vi "HDF5_append-dataset-Test6vi.vi"() -> ()   [LabVIEW 2018]
uses:
  <vilib>/addons/h5labview2/file/H5F.lvlib
  <vilib>/addons/h5labview2/file/H5Fmode.ctl
  <vilib>/addons/h5labview2/dataset/H5D.lvlib
  HDF5/HDF5_ToneInfoClust.ctl
  <vilib>/addons/h5labview2/dataset/H5Dwrite.llb/H5Dwrite.xnode
  <vilib>/addons/h5labview2/space/H5S.lvlib
  <vilib>/addons/h5labview2/base/H5Equery.vi
  HDF5/lib_path_mod_20200519.vi
  <vilib>/addons/h5labview2/dataset/H5Dread.llb/H5Dread.xnode
  HDF5/HDF5_ToneInfoZoomAryClust.ctl
  <vilib>/addons/h5labview2/base/hid_t_renamed.ctl
panel:
  out "Tone2":T1[](array[typedef])
  out "Tone1":T1[](array[typedef])
  in  "data":i32[][](array[numeric])=[[0, 1, 2, 3, 4], [5, 6, 7, 8, 9]]
  out "ms/append":dbl
  out "timer (ms)":u32
  out "progress":i32(slide)=9999 scale=0.0..10000.0
  in  "repetitions":i32=10
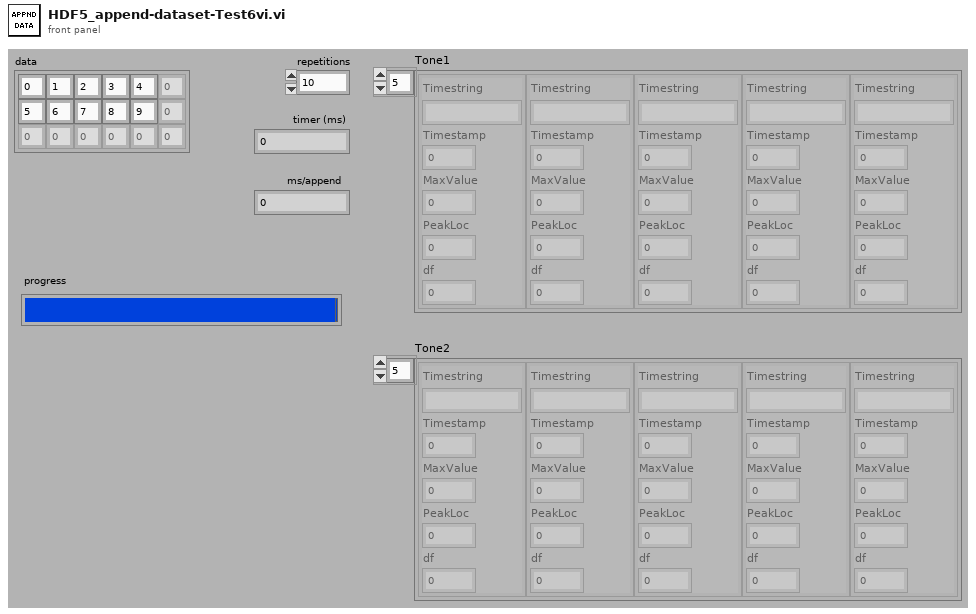
[diagram p1: front panel]
types:
  T1 = typedef "HDF5_ToneInfoClust.ctl" = cluster{"Timestring":string, "Timestamp":dbl, "MaxValue":dbl, "PeakLoc":dbl, "df":dbl}
  T2 = typedef "H5F.lvlib/H5Fmode.ctl" = enum16{"read-only", "read-write", "overwrite", "create new", "open or create"}
  T3 = typedef "HDF5_ToneInfoZoomAryClust.ctl" = cluster{"Timestring":string, "Timestamp":timestamp, "MaxValue":dbl, "PeakLoc":dbl, "df":dbl, "Zoom":dbl[]}
  T4 = typedef "HDF5_ToneInfoClust.ctl" = cluster{"Timestring":string, "Timestamp":timestamp, "MaxValue":dbl, "PeakLoc":dbl, "df":dbl}
  T5 = typedef "hid_t.ctl" = i32
  T6 = typedef "hid_t_renamed.ctl" = i32
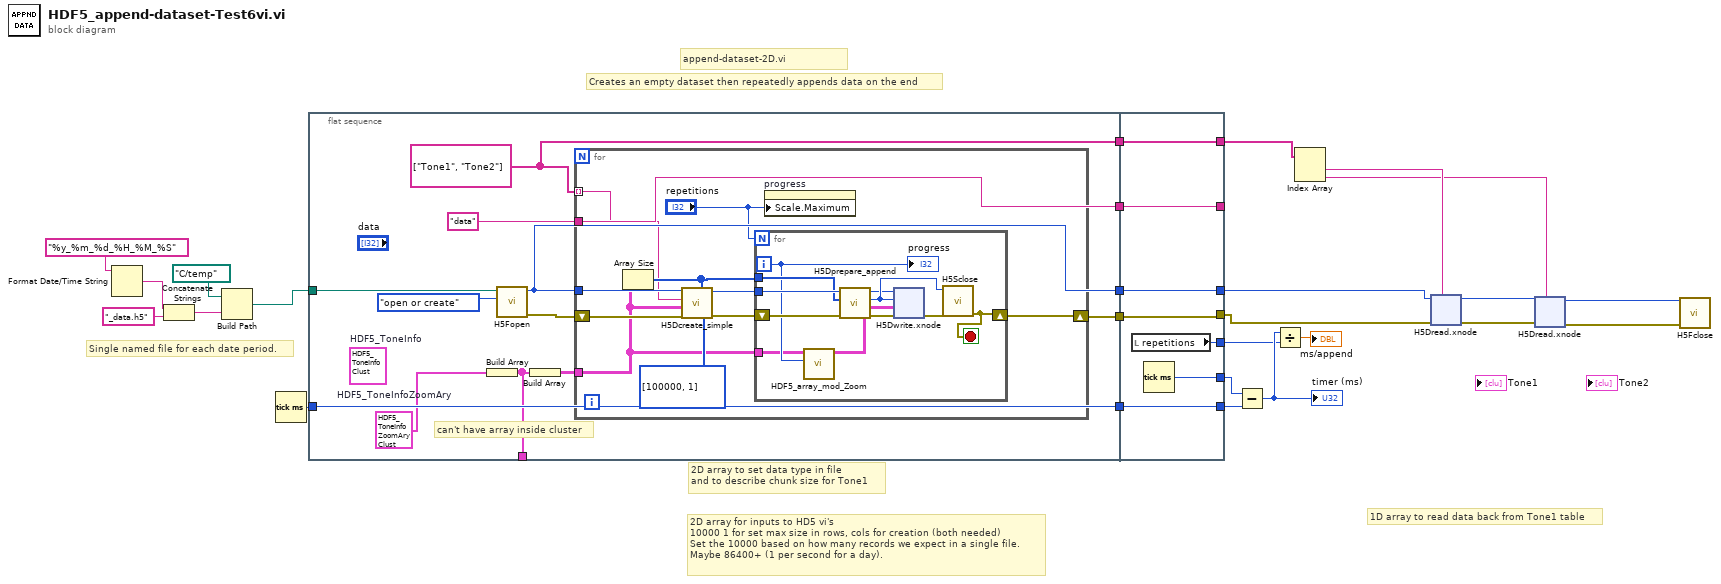
[diagram p0: block diagram]
diagram:
  # "2D array to set data type in file\nand to describe chunk size for Tone1"
  # "1D array to read data back from Tone1 table"
  # "2D array for inputs to HD5 vi's\n10000 1 for set max size in rows, cols for creation (both needed) \nSet the 10000 based on how many records we expect in a single file.\nMaybe 86400+ (1 per second for a day)."
  # "Single named file for each date period."
  # "Creates an empty dataset then repeatedly appends data on the end"
  # "append-dataset-2D.vi"
  n1 = Format Date/Time String(time format string (%c)="%y_%m_%d_%H_%M_%S") -> (date/time string=w17:string)  [unwired: 2 in]
  n2 = Concatenate Strings(w17, "_data.h5" ("string")) -> (w19:string)
  n3 = Build Path(base path=path "C:/temp", name or relative path=w19) -> (appended path=w15:path)
  n4 = Tick Count (ms)() -> (millisecond timer value=w27:u32)
  n5 = flat-sequence {
    tunnel: w27 -> [w36]
    tunnel: [w36] -> w26
    tunnel: w15 -> [w35]
    tunnel: [w33] -> w13
    tunnel: [w32] -> w12
    tunnel: [w31] -> w1
    tunnel: [w30] -> w11
    tunnel: [w29] -> w9
    tunnel: w26 -> [w84]
    tunnel: [w85] -> w25
    tunnel: [w84] -> w24
    tunnel: [w83] -> w22
    tunnel: [w82] -> w14
    tunnel: w13 -> [w82]
    tunnel: [w81] -> _
    tunnel: w12 -> [w81]
    tunnel: [w80] -> w10
    tunnel: w11 -> [w80]
    tunnel: w9 -> [w79]
    tunnel: [w79] -> w7
    frame #0 {
      w28 = T3 {"Timestring"="Timestamp string goes here", "Timestamp"=timestamp(0 s since 1904-01-01), "MaxValue"=0.0, "PeakLoc"=0.0, "df"=0.0, "Zoom"=[0.0, 0.0, 0.0, 0.0, 0.0, 0.0, 0.0, 0.0, 0.0, 0.0, 0.0, 0.0, 0.0, 0.0, 0.0, 0.0, 0.0, 0.0, 0.0, 0.0, 0.0, 0.0, 0.0, 0.0, 0.0, 0.0, 0.0, 0.0, 0.0, 0.0, 0.0, 0.0, 0.0, 0.0, 0.0, 0.0, 0.0, 0.0, 0.0, 0.0, 0.0, 0.0, 0.0, 0.0, 0.0, 0.0, 0.0, 0.0, 0.0, 0.0, 0.0, 0.0, 0.0, 0.0, 0.0, 0.0, 0.0, 0.0, 0.0, 0.0, 0.0, 0.0, 0.0, 0.0, 0.0, 0.0, 0.0, 0.0, 0.0, 0.0, 0.0, 0.0, 0.0, 0.0, 0.0, 0.0, 0.0, 0.0, 0.0, 0.0, 0.0, 0.0, 0.0, 0.0, 0.0, 0.0, 0.0, 0.0, 0.0, 0.0, 0.0, 0.0, 0.0, 0.0, 0.0, 0.0, 0.0, 0.0, 0.0, 0.0, 0.0, 0.0, 0.0, 0.0, 0.0, 0.0, 0.0, 0.0, 0.0, 0.0, 0.0, 0.0, 0.0, 0.0, 0.0, 0.0, 0.0, 0.0, 0.0, 0.0, 0.0, 0.0, 0.0, 0.0, 0.0, 0.0, 0.0, 0.0, 0.0, 0.0, 0.0, 0.0, 0.0, 0.0, 0.0, 0.0, 0.0, 0.0, 0.0, 0.0, 0.0, 0.0, 0.0, 0.0, 0.0, 0.0, 0.0, 0.0, 0.0, 0.0, 0.0, 0.0, 0.0, 0.0, 0.0, 0.0, 0.0, 0.0, 0.0, 0.0, 0.0, 0.0, 0.0, 0.0, 0.0, 0.0, 0.0, 0.0, 0.0, 0.0, 0.0, 0.0, 0.0, 0.0, 0.0, 0.0, 0.0, 0.0, 0.0, 0.0, 0.0, 0.0, 0.0, 0.0, 0.0, 0.0, 0.0, 0.0, 0.0, 0.0, 0.0, 0.0, 0.0, 0.0, 0.0, 0.0, 0.0, 0.0, 0.0, 0.0, 0.0, 0.0, 0.0, 0.0, 0.0, 0.0, 0.0, 0.0, 0.0, 0.0, 0.0, 0.0, 0.0, 0.0, 0.0, 0.0, 0.0, 0.0, 0.0, 0.0, 0.0, 0.0, 0.0, 0.0, 0.0, 0.0, 0.0, 0.0, 0.0, 0.0, 0.0, 0.0, 0.0, 0.0, 0.0, 0.0, 0.0, 0.0, 0.0, 0.0, 0.0, 0.0, 0.0, 0.0, 0.0, 0.0, 0.0, 0.0, 0.0, 0.0, 0.0, 0.0, 0.0, 0.0, 0.0, 0.0, 0.0, 0.0, 0.0, 0.0, 0.0, 0.0, 0.0, 0.0, 0.0, 0.0, 0.0, 0.0, 0.0, 0.0, 0.0, 0.0, 0.0, 0.0, 0.0, 0.0, 0.0, 0.0, 0.0, 0.0, 0.0, 0.0, 0.0, 0.0, 0.0, 0.0, 0.0, 0.0, 0.0, 0.0, 0.0, 0.0, 0.0, 0.0, 0.0, 0.0, 0.0, 0.0, 0.0, 0.0, 0.0, 0.0, 0.0, 0.0, 0.0, 0.0, 0.0, 0.0, 0.0, 0.0, 0.0, 0.0, 0.0, 0.0, 0.0, 0.0, 0.0, 0.0, 0.0, 0.0, 0.0, 0.0, 0.0, 0.0, 0.0, 0.0, 0.0, 0.0, 0.0, 0.0, 0.0, 0.0, 0.0, 0.0, 0.0, 0.0, 0.0, 0.0, 0.0, 0.0, 0.0, 0.0, 0.0, 0.0, 0.0, 0.0, 0.0, 0.0, 0.0, 0.0, 0.0, 0.0, 0.0, 0.0, 0.0, 0.0, 0.0, 0.0, 0.0, 0.0, 0.0, 0.0, 0.0, 0.0, 0.0, 0.0, 0.0, 0.0, 0.0, 0.0, 0.0, 0.0, 0.0, 0.0, 0.0, 0.0, 0.0, 0.0, 0.0, 0.0, 0.0, 0.0, 0.0, 0.0, 0.0, 0.0, 0.0, 0.0, 0.0, 0.0, 0.0, 0.0, 0.0, 0.0, 0.0, 0.0, 0.0, 0.0, 0.0, 0.0, 0.0, 0.0, 0.0, 0.0, 0.0, 0.0, 0.0, 0.0, 0.0, 0.0, 0.0, 0.0, 0.0, 0.0, 0.0, 0.0, 0.0, 0.0, 0.0, 0.0, 0.0, 0.0, 0.0, 0.0, 0.0, 0.0, 0.0, 0.0, 0.0, 0.0, 0.0, 0.0, 0.0, 0.0, 0.0, 0.0, 0.0, 0.0, 0.0, 0.0, 0.0, 0.0, 0.0, 0.0, 0.0, 0.0, 0.0, 0.0, 0.0, 0.0, 0.0, 0.0, 0.0, 0.0, 0.0, 0.0, 0.0, 0.0, 0.0, 0.0, 0.0, 0.0, 0.0, 0.0, 0.0, 0.0, 0.0, 0.0, 0.0, 0.0, 0.0, 0.0, 0.0, 0.0, 0.0, 0.0, 0.0, 0.0, 0.0, 0.0, 0.0, 0.0, 0.0, 0.0, 0.0, 0.0, 0.0, 0.0, 0.0, 0.0, 0.0, 0.0, 0.0, 0.0, 0.0, 0.0, 0.0, 0.0, 0.0, 0.0, 0.0, 0.0, 0.0, 0.0, 0.0, 0.0, 0.0, 0.0, 0.0, 0.0, 0.0, 0.0, 0.0, 0.0, 0.0, 0.0, 0.0, 0.0, 0.0, 0.0, 0.0, 0.0, 0.0, 0.0, 0.0, 0.0, 0.0, 0.0, 0.0, 0.0, 0.0, 0.0, 0.0, 0.0, 0.0, 0.0, 0.0, 0.0, 0.0, 0.0, 0.0, 0.0, 0.0, 0.0, 0.0, 0.0, 0.0, 0.0, 0.0, 0.0, 0.0, 0.0, 0.0, 0.0, 0.0, 0.0, 0.0, 0.0, 0.0, 0.0, 0.0, 0.0, 0.0, 0.0, 0.0, 0.0, 0.0, 0.0, 0.0, 0.0, 0.0, 0.0, 0.0, 0.0, 0.0, 0.0, 0.0, 0.0, 0.0, 0.0, 0.0, 0.0, 0.0, 0.0, 0.0, 0.0, 0.0, 0.0, 0.0, 0.0, 0.0, 0.0, 0.0, 0.0, 0.0, 0.0, 0.0, 0.0, 0.0, 0.0, 0.0, 0.0, 0.0, 0.0, 0.0, 0.0, 0.0, 0.0, 0.0, 0.0, 0.0, 0.0, 0.0, 0.0, 0.0, 0.0, 0.0, 0.0, 0.0, 0.0, 0.0, 0.0, 0.0, 0.0, 0.0, 0.0, 0.0, 0.0, 0.0, 0.0, 0.0, 0.0, 0.0, 0.0, 0.0, 0.0, 0.0, 0.0, 0.0, 0.0, 0.0, 0.0, 0.0, 0.0, 0.0, 0.0, 0.0, 0.0, 0.0, 0.0, 0.0, 0.0, 0.0, 0.0, 0.0, 0.0, 0.0, 0.0, 0.0, 0.0, 0.0, 0.0, 0.0, 0.0, 0.0, 0.0, 0.0, 0.0, 0.0, 0.0, 0.0, 0.0, 0.0, 0.0, 0.0, 0.0, 0.0, 0.0, 0.0, 0.0, 0.0, 0.0, 0.0, 0.0, 0.0, 0.0, 0.0, 0.0, 0.0, 0.0, 0.0, 0.0, 0.0, 0.0, 0.0, 0.0, 0.0, 0.0, 0.0, 0.0, 0.0, 0.0, 0.0, 0.0, 0.0, 0.0, 0.0, 0.0, 0.0, 0.0, 0.0, 0.0, 0.0, 0.0, 0.0, 0.0, 0.0, 0.0, 0.0, 0.0, 0.0, 0.0, 0.0, 0.0, 0.0, 0.0, 0.0, 0.0, 0.0, 0.0, 0.0, 0.0, 0.0, 0.0, 0.0, 0.0, 0.0, 0.0, 0.0, 0.0, 0.0, 0.0, 0.0, 0.0, 0.0, 0.0, 0.0, 0.0, 0.0, 0.0, 0.0, 0.0, 0.0, 0.0, 0.0, 0.0, 0.0, 0.0, 0.0, 0.0, 0.0, 0.0, 0.0, 0.0, 0.0, 0.0, 0.0, 0.0, 0.0, 0.0, 0.0, 0.0, 0.0, 0.0, 0.0, 0.0, 0.0, 0.0, 0.0, 0.0, 0.0, 0.0, 0.0, 0.0, 0.0, 0.0, 0.0, 0.0, 0.0, 0.0, 0.0, 0.0, 0.0, 0.0, 0.0, 0.0, 0.0, 0.0, 0.0, 0.0, 0.0, 0.0, 0.0, 0.0, 0.0, 0.0, 0.0, 0.0, 0.0, 0.0, 0.0, 0.0, 0.0, 0.0, 0.0, 0.0, 0.0, 0.0, 0.0, 0.0, 0.0, 0.0, 0.0, 0.0, 0.0, 0.0, 0.0, 0.0, 0.0, 0.0, 0.0, 0.0, 0.0, 0.0, 0.0, 0.0, 0.0, 0.0, 0.0, 0.0, 0.0, 0.0, 0.0, 0.0, 0.0, 0.0, 0.0, 0.0, 0.0, 0.0, 0.0, 0.0, 0.0, 0.0, 0.0, 0.0, 0.0, 0.0, 0.0, 0.0, 0.0, 0.0, 0.0, 0.0, 0.0, 0.0, 0.0, 0.0, 0.0, 0.0, 0.0, 0.0, 0.0, 0.0, 0.0, 0.0, 0.0, 0.0, 0.0, 0.0, 0.0, 0.0, 0.0, 0.0, 0.0, 0.0, 0.0, 0.0, 0.0, 0.0, 0.0, 0.0, 0.0, 0.0, 0.0, 0.0, 0.0, 0.0, 0.0, 0.0, 0.0, 0.0, 0.0, 0.0, 0.0, 0.0, 0.0, 0.0, 0.0, 0.0, 0.0, 0.0, 0.0, 0.0, 0.0, 0.0, 0.0, 0.0, 0.0, 0.0, 0.0, 0.0, 0.0, 0.0, 0.0, 0.0, 0.0, 0.0, 0.0, 0.0, 0.0, 0.0, 0.0, 0.0, 0.0, 0.0, 0.0, 0.0, 0.0, 0.0, 0.0, 0.0, 0.0, 0.0, 0.0, 0.0, 0.0, 0.0, 0.0, 0.0, 0.0, 0.0, 0.0, 0.0, 0.0, 0.0, 0.0, 0.0, 0.0, 0.0, 0.0, 0.0, 0.0, 0.0, 0.0, 0.0, 0.0, 0.0, 0.0, 0.0, 0.0, 0.0, 0.0, 0.0, 0.0, 0.0, 0.0, 0.0, 0.0, 0.0, 0.0, 0.0, 0.0, 0.0, 0.0, 0.0, 0.0, 0.0, 0.0, 0.0, 0.0, 0.0, 0.0, 0.0, 0.0, 0.0, 0.0, 0.0, 0.0, 0.0, 0.0, 0.0, 0.0, 0.0, 0.0, 0.0, 0.0, 0.0, 0.0, 0.0, 0.0, 0.0, 0.0, 0.0, 0.0, 0.0, 0.0, 0.0, 0.0, 0.0, 0.0, 0.0, 0.0, 0.0]}  # HDF5_ToneInfoZoomAry
      w29 = string[] ["Tone1", "Tone2"]
      (unwired) T4 {"Timestring"="Timestamp string goes here", "Timestamp"=timestamp(0 s since 1904-01-01), "MaxValue"=0.0, "PeakLoc"=0.0, "df"=0.0}  # HDF5_ToneInfo
      w32 = "data" ("name")
      # "can't have array inside cluster"
      n6 = Build Array(w28) -> (w31:T3[])
      n7 = call <vilib>:"H5Fopen.vi"("mode (read-only)"=H5Fmode."open or create" ("mode"), "path"=w35) -> ("error out"=w37:errorcluster, "ref out"=w33:T5)  [unwired: 8 in]
      n8 = Build Array(w31) -> (w34:T3[][])
      n9 = for {
        tunnel: w34 -> [w39]
        tunnel: w33 -> [w43]
        tunnel: w32 -> [_]
        shift-right: [w42] -> w30
        shift-left: w37 -> [w46]
        tunnel: w29 -> [w41] mode=indexing
        n10 = Array Size(array=w39) -> (size(s)=w44:i32[])
        n11 = call <vilib>:"H5Dcreate_simple.vi"("max size"=u64[] [100000, 1], "chunk size"=w44, "error in (no error)"=w46, "type in"=w39, "name"=w41, "ref in"=w43) -> ("error out"=w47:errorcluster, "dset out"=w48:T5)  [unwired: 4 in]
        n12 = for {
          N: "repetitions" -> [_]
          shift-right: [w55] -> w42
          shift-left: w47 -> [w56]
          tunnel: w44 -> [w57]
          tunnel: w48 -> [w58]
          tunnel: w39 -> [w50]
          i -> [w51]
          stop <- w55 stop-if-true
          n13 = call "HDF5_array_mod_Zoom.vi"("delta"=w51, "Array in"=w50) -> ("Array out"=w49:T3[][])  [unwired: 9 in]
          n14 = call <vilib>:"H5Dprepare_append.vi"("error in (no error)"=w56, "append dims"=w57, "dset in"=w58) -> ("error out"=w59:errorcluster, "space out"=w53:T5, "dset out"=w52:T5)  [unwired: 5 in, 1 out]
          n15 = xnode "H5Dwrite.xnode"("error in (no error)"=w59, "data"=w49, "file space"=w53, "ref in"=w52) -> ("error out"=w54:errorcluster)  [unwired: 3 in, 2 out]
          n16 = call <vilib>:"H5Sclose.vi"("error in (no error)"=w54, "space in"=w53) -> ("error out"=w55:errorcluster)  [unwired: 9 in]
          "progress" <- w51
        }
        n17 = property on="progress" class="Slide (strict)"("Scale.Maximum"="repetitions") -> ()  [unwired: 2 in, 2 out]
      }
    }
    frame #1 {
      n18 = local read "repetitions"() -> (w83:i32)
      n19 = Tick Count (ms)() -> (millisecond timer value=w85:u32)
    }
  }
  n20 = Subtract(x=w25, y=w24) -> (x-y=w23:u32)
  "timer (ms)" <- w23
  n21 = Divide(x=w23, y=w22) -> (x/y=→"ms/append":dbl)
  n22 = Index Array(array=w7) -> (element #1=w6:string, element #2=w5:string)  [unwired: 2 in]
  n23 = xnode "H5Dread.xnode"("dataset name (this)"=w6, "error in (no error)"=w10, "ref in"=w14) -> ("error out"=w4:errorcluster, "ref out"=w8:i32)  [unwired: 3 in, 2 out]
  n24 = xnode "H5Dread.xnode"("dataset name (this)"=w5, "error in (no error)"=w4, "ref in"=w8) -> ("error out"=w2:errorcluster, "ref out"=w3:T6)  [unwired: 3 in, 2 out]
  n25 = call <vilib>:"H5Fclose.vi"("error in (no error)"=w2, "ref"=w3) -> ()  [unwired: 9 in, 1 out]
